vi "temp.vi"() -> ()   [LabVIEW 2016]
uses:
  <vilib>/NXT/Block Support/NXT_OutputPort.ctl
  <vilib>/NXT/NXTIO Xnodes/NXTIONodeSubVIs/LEGOMoveAllMotors.vi
  <vilib>/NXT/Dual Mode Library/Sensors/EV3_Color_Reflect.vi
  <vilib>/NXT/Dual Mode Library/Waits/Wait_Num.vi
  <vilib>/NXT/NXTIO Xnodes/NXTIONodeSubVIs/NXTMotorRunDistance.vi
  <vilib>/NXT/NXTIO Xnodes/NXTIONodeSubVIs/LEGOStopAllMotors.vi
  <vilib>/NXT/Subs/LVHSConnector.ctl
  <vilib>/NXT/NXTIO Xnodes/NXTIOXNode/NXTIO.xnode
  <vilib>/NXT/NXTIO Xnodes/AddressXNode/NXTIOAddress.xnode
  <vilib>/NXT/LegoClasses/BrickReference/BrickReference.lvclass
panel:
  out "Numeric 2":dbl
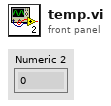
[diagram p1: front panel]
types:
  T1 = typedef "LVHSConnector.ctl" = refnum<class "BrickReference.lvclass">
  T2 = typedef "NXT_OutputPort.ctl" = u8
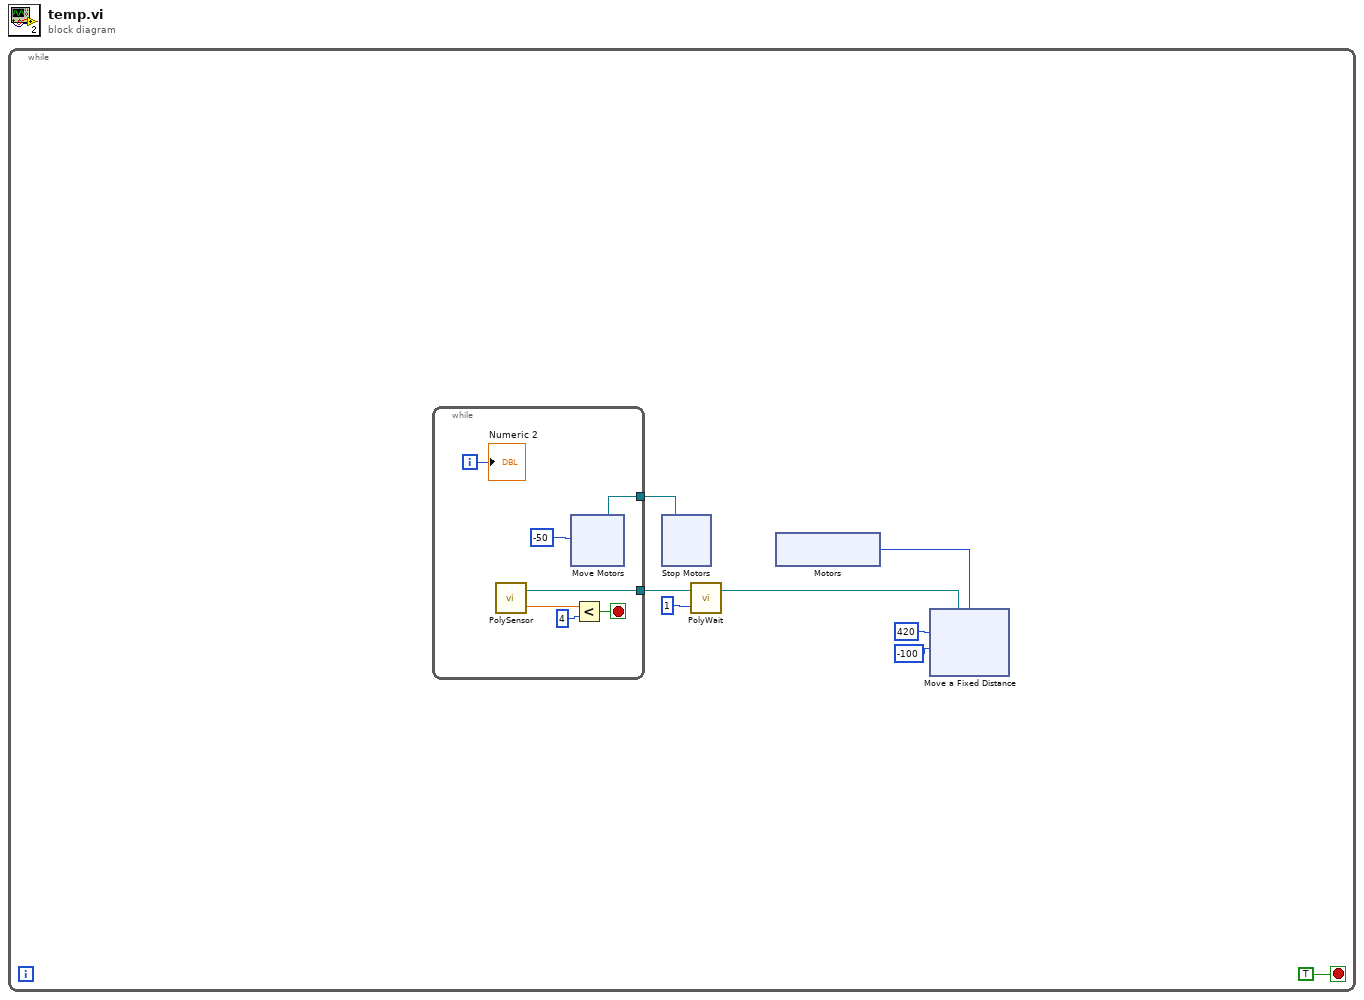
[diagram p0: block diagram]
diagram:
  n1 = while {
    stop <- TRUE stop-if-true
    n2 = while {
      tunnel: [w28] -> w5
      tunnel: [w27] -> w3
      i -> [w29]
      stop <- w31 stop-if-true
      n3 = call-poly <vilib>:"PolySensor.vi"() -> ("Scaled Value"=w26:sgl, "NXT/EV3"=w28:T1)  [unwired: 3 in]
      n4 = xnode "Move Motors"("Power/Speed 1"=-50) -> ("NXT/EV3"=w27:T1)  [unwired: 2 in]
      n5 = Less?(x=w26, y=4) -> (x < y?=w31:bool)
      "Numeric 2" <- w29
    }
    n6 = xnode "Stop Motors"("NXT/EV3"=w3) -> ()  [unwired: 1 in, 1 out]
    n7 = call-poly <vilib>:"PolyWait.vi"("Time (1 sec)"=1, "NXT/EV3"=w5) -> ("NXT/EV3"=w1:T1)  [unwired: 2 in]
    n8 = xnode "Motors"() -> ("Motor"=w6:T2)
    n9 = xnode "Move a Fixed Distance"("Speed 1"=-100, "Distance 1"=420, "Motors"=w6, "NXT/EV3"=w1) -> ()  [unwired: 1 out]
  }
